vi "Session6_StateMachine_Internal_Event.vi"() -> ()   [LabVIEW 2016]
uses:
  EnuStateType.ctl
panel:
  in  "log":bool
  in  "Timeout":i32=1
  out "Loop Counter 2":i32
  out "Loop Counter 1":i32
  out "Thermometer":dbl(slide) scale=0.0..100.0
  out "Temp Value":dbl
  in  "Clear":bool
  out "Temp Chart":dbl(graph)
  in  "Sensor Simulator":dbl(slide) scale=0.0..100.0
  in  "stop":bool
  # "Session 5 – Project: State Machine Extended Discussion"
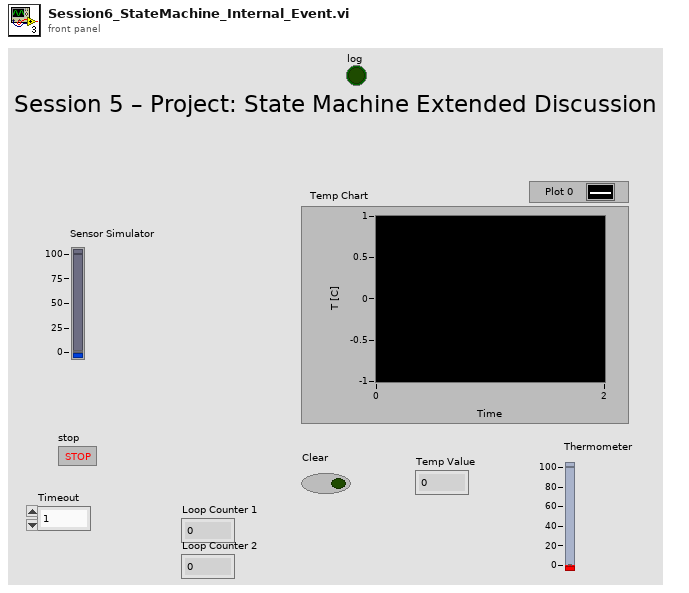
[diagram p1: front panel]
types:
  T1 = typedef "EnuStateType.ctl" = enum16{"Initialize", "IDLE", "Clear Chart", "Update Chart", "Save"}
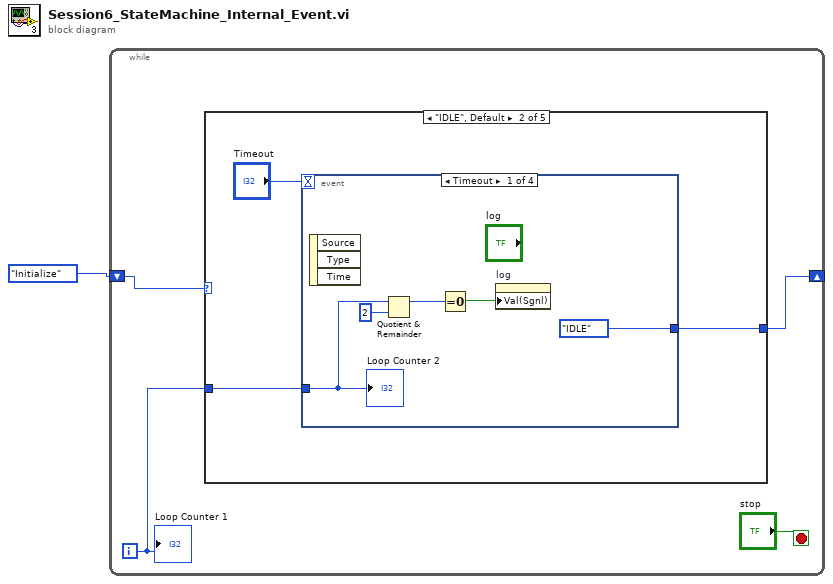
[diagram p0: block diagram]
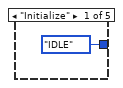
[diagram p2: hidden frame]
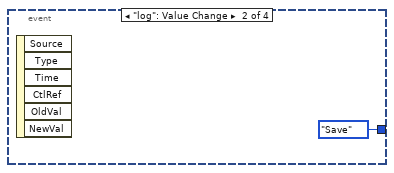
[diagram p3: hidden frame]
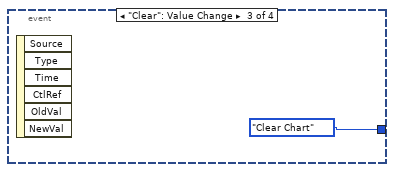
[diagram p4: hidden frame]
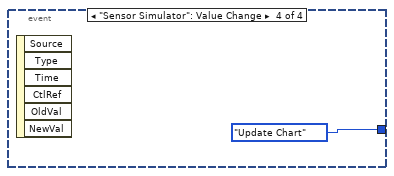
[diagram p5: hidden frame]
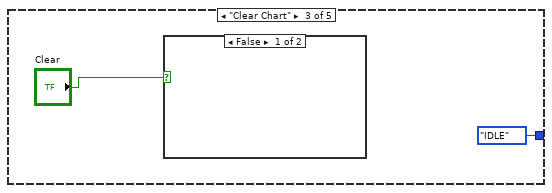
[diagram p6: hidden frame]
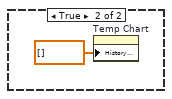
[diagram p7: hidden frame]
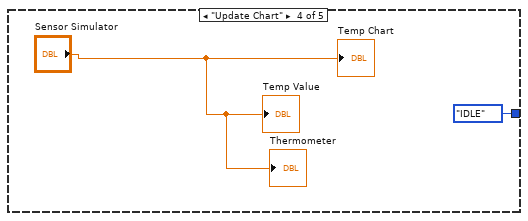
[diagram p8: hidden frame]
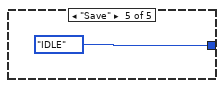
[diagram p9: hidden frame]
diagram:
  n1 = while {
    shift-right: [w2] -> _
    shift-left: EnuStateType."Initialize" -> [w4]
    i -> [w3]
    stop <- "stop" stop-if-true
    n2 = case shown="\"IDLE\", Default" w4 {
      tunnel: w3 -> [_ w8 _ _ _]
      tunnel: [EnuStateType."IDLE" w7 EnuStateType."IDLE" EnuStateType."IDLE" EnuStateType."IDLE"] -> w2
      frame "Initialize" {
      }
      frame "IDLE", Default {
        n3 = event shown="[0] Timeout" {
          selector: _ -> [_ _ _ _]
          dyn-events: _ -> [_ _ _ _]
          timeout: "Timeout" -> [_ _ _ _]
          tunnel: w8 -> [w13 _ _ _]
          tunnel: [EnuStateType."IDLE" EnuStateType."Save" EnuStateType."Clear Chart" EnuStateType."Update Chart"] -> w7
          event Timeout {
            n4 = event-data() -> ()  [unwired: 1 in, 3 out]
            n5 = Quotient & Remainder(x=w13, y=2) -> (x-y*floor(x/y)=w11:i32)  [unwired: 1 out]
            n6 = Equal To 0?(x=w11) -> (x = 0?=w10:bool)
            n7 = property on="log" class="Bool (strict)"("Val(Sgnl)"=w10) -> ()  [unwired: 2 in, 2 out]
            "Loop Counter 2" <- w13
          }
          event "log": Value Change {
            n8 = event-data() -> ()  [unwired: 1 in, 6 out]
          }
          event "Clear": Value Change {
            n9 = event-data() -> ()  [unwired: 1 in, 6 out]
          }
          event "Sensor Simulator": Value Change {
            n10 = event-data() -> ()  [unwired: 1 in, 6 out]
          }
        }
      }
      frame "Clear Chart" {
        n11 = case shown="False" "Clear" {
          frame False {
          }
          frame True {
            n12 = property on="Temp Chart" class="WFChart (strict)"("History Data"=dbl[] []) -> ()  [unwired: 2 in, 2 out]
          }
        }
      }
      frame "Update Chart" {
        "Temp Chart" <- "Sensor Simulator"
        "Temp Value" <- "Sensor Simulator"
        "Thermometer" <- "Sensor Simulator"
      }
      frame "Save" {
      }
    }
    "Loop Counter 1" <- w3
  }
